vi "ZCAN_ReceiveData_2.vi"() -> ()   [LabVIEW 2020]
uses:
  data_type/ZCANDataObj.ctl
  bin/zlgcan_wrap.dll
panel:
  in  "type of receipt":enum16{"CAN", "CANFD", "合并接收"}(ring)=enum."合并接收"
  out "error out":errorcluster caption="错误输出"
  out "Receive_Num":u32
  in  "can_handle":u32
  in  "error in (no error)":errorcluster caption="错误输入（无错误）"
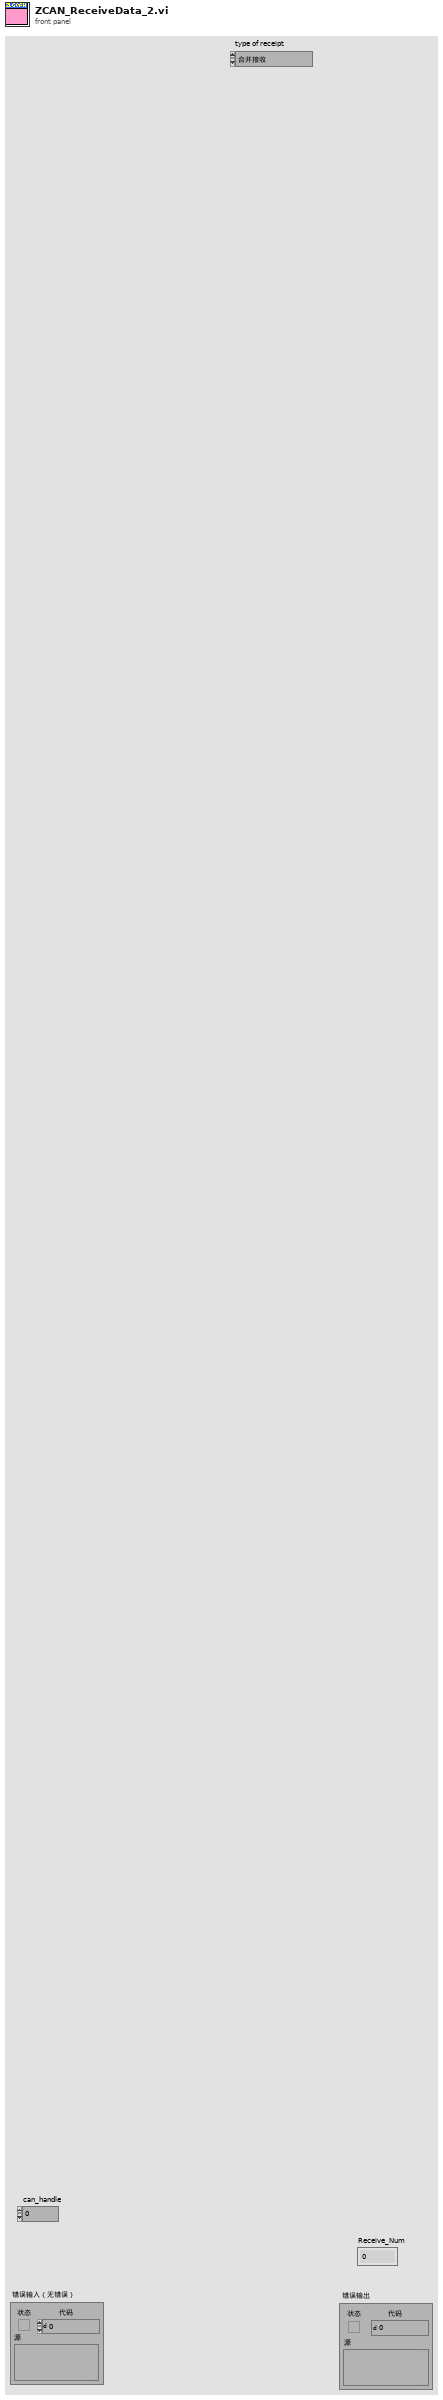
[diagram p1: front panel]
types:
  T1 = typedef "zlgcan.lvlib/ZCANDataObj.ctl" = cluster{"Data_Type":u8, "CAN_CH":u8, "rawVal(未使用)":u16, "extraData[4]（未使用）":cluster{"[0]":u8, "[1]":u8, "[2]":u8, "[3]":u8}, "canCANFDData":cluster{"时间戳+混合标志位":cluster{"时间戳":u64, "混合标志位":u32}, "extraData[4]（未使用）":cluster{"[0]":u8, "[1]":u8, "[2]":u8, "[3]":u8}, "frame":cluster{"can_id":u32, "Data长度":u8, "CANFD加速？":u8, "__res0":u8, "__res1":u8, "data":cluster{"CANData[0]":u8, "CANData[1]":u8, "CANData[2]":u8, "CANData[3]":u8, "CANData[4]":u8, "CANData[5]":u8, "CANData[6]":u8, "CANData[7]":u8, "CANData[8]":u8, "CANData[9]":u8, "CANData[10]":u8, "CANData[11] ":u8, "CANData[12] ":u8, "CANData[13] ":u8, "CANData[14] ":u8, "CANData[15] ":u8, "CANData[16]":u8, "CANData[17]":u8, "CANData[18]":u8, "CANData[19]":u8, "CANData[20]":u8, "CANData[21]":u8, "CANData[22]":u8, "CANData[23]":u8, "CANData[24] ":u8, "CANData[25]":u8, "CANData[26]":u8, "CANData[27]":u8, "CANData[28]":u8, "CANData[29]":u8, "CANData[30]":u8, "CANData[31]":u8, "CANData[32]":u8, "CANData[33]":u8, "CANData[34]":u8, "CANData[35]":u8, "CANData[36]":u8, "CANData[37]":u8, "CANData[38]":u8, "CANData[39]":u8, "CANData[40]":u8, "CANData[41]":u8, "CANData[42]":u8, "CANData[43]":u8, "CANData[44]":u8, "CANData[45]":u8, "CANData[46]":u8, "CANData[47]":u8, "CANData[48]":u8, "CANData[49]":u8, "CANData[50]":u8, "CANData[51]":u8, "CANData[52]":u8, "CANData[53]":u8, "CANData[54]":u8, "CANData[55]":u8, "CANData[56]":u8, "CANData[57]":u8, "CANData[58]":u8, "CANData[59]":u8, "CANData[60]":u8, "CANData[61]":u8, "CANData[62]":u8, "CANData[63]":u8}}}, "raw":cluster{"[0]":u8, "[1]":u8, "[2]":u8, "[3]":u8, "[4]":u8, "[5]":u8, "[6]":u8, "[7]":u8, "[8]":u8, "[9]":u8, "[10]":u8, "[11]":u8, "[12]":u8, "[13]":u8, "[14]":u8, "[15]":u8, "[16]":u8, "[17]":u8, "[18]":u8, "[19]":u8, "[20]":u8, "[21]":u8, "[22]":u8, "[23]":u8, "[24]":u8, "[25]":u8, "[26]":u8, "[27]":u8, "[28]":u8, "[29]":u8, "[30]":u8, "[31]":u8, "[32]":u8, "[33]":u8, "[34]":u8, "[35]":u8, "[36]":u8, "[37]":u8, "[38]":u8, "[39]":u8, "[40]":u8, "[41]":u8, "[42]":u8, "[43]":u8, "[44]":u8, "[45]":u8, "[46]":u8, "[47]":u8, "[48]":u8, "[49]":u8, "[50]":u8, "[51]":u8, "[52]":u8, "[53]":u8, "[54]":u8, "[55]":u8, "[56]":u8, "[57]":u8, "[58]":u8, "[59]":u8, "[60]":u8, "[61]":u8, "[62]":u8, "[63]":u8, "[64]":u8, "[65]":u8, "[73]":u8, "[72]":u8, "[71]":u8, "[70]":u8, "[69]":u8, "[68]":u8, "[67]":u8, "[66]":u8, "[74]":u8, "[75]":u8, "[83]":u8, "[82]":u8, "[81]":u8, "[80]":u8, "[79]":u8, "[78]":u8, "[77]":u8, "[76]":u8, "[84]":u8, "[85]":u8, "[91]":u8, "[90]":u8, "[89]":u8, "[88]":u8, "[87]":u8, "[86]":u8}}
  T2 = cluster{"时间戳+混合标志位":cluster{"时间戳":u64, "混合标志位":u32}, "extraData[4]（未使用）":cluster{"[0]":u8, "[1]":u8, "[2]":u8, "[3]":u8}, "frame":cluster{"can_id":u32, "Data长度":u8, "CANFD加速？":u8, "__res0":u8, "__res1":u8, "data":cluster{"CANData[0]":u8, "CANData[1]":u8, "CANData[2]":u8, "CANData[3]":u8, "CANData[4]":u8, "CANData[5]":u8, "CANData[6]":u8, "CANData[7]":u8, "CANData[8]":u8, "CANData[9]":u8, "CANData[10]":u8, "CANData[11] ":u8, "CANData[12] ":u8, "CANData[13] ":u8, "CANData[14] ":u8, "CANData[15] ":u8, "CANData[16]":u8, "CANData[17]":u8, "CANData[18]":u8, "CANData[19]":u8, "CANData[20]":u8, "CANData[21]":u8, "CANData[22]":u8, "CANData[23]":u8, "CANData[24] ":u8, "CANData[25]":u8, "CANData[26]":u8, "CANData[27]":u8, "CANData[28]":u8, "CANData[29]":u8, "CANData[30]":u8, "CANData[31]":u8, "CANData[32]":u8, "CANData[33]":u8, "CANData[34]":u8, "CANData[35]":u8, "CANData[36]":u8, "CANData[37]":u8, "CANData[38]":u8, "CANData[39]":u8, "CANData[40]":u8, "CANData[41]":u8, "CANData[42]":u8, "CANData[43]":u8, "CANData[44]":u8, "CANData[45]":u8, "CANData[46]":u8, "CANData[47]":u8, "CANData[48]":u8, "CANData[49]":u8, "CANData[50]":u8, "CANData[51]":u8, "CANData[52]":u8, "CANData[53]":u8, "CANData[54]":u8, "CANData[55]":u8, "CANData[56]":u8, "CANData[57]":u8, "CANData[58]":u8, "CANData[59]":u8, "CANData[60]":u8, "CANData[61]":u8, "CANData[62]":u8, "CANData[63]":u8}}}
  T3 = cluster{"can_id":u32, "Data长度":u8, "CANFD加速？":u8, "__res0":u8, "__res1":u8, "data":cluster{"CANData[0]":u8, "CANData[1]":u8, "CANData[2]":u8, "CANData[3]":u8, "CANData[4]":u8, "CANData[5]":u8, "CANData[6]":u8, "CANData[7]":u8, "CANData[8]":u8, "CANData[9]":u8, "CANData[10]":u8, "CANData[11] ":u8, "CANData[12] ":u8, "CANData[13] ":u8, "CANData[14] ":u8, "CANData[15] ":u8, "CANData[16]":u8, "CANData[17]":u8, "CANData[18]":u8, "CANData[19]":u8, "CANData[20]":u8, "CANData[21]":u8, "CANData[22]":u8, "CANData[23]":u8, "CANData[24] ":u8, "CANData[25]":u8, "CANData[26]":u8, "CANData[27]":u8, "CANData[28]":u8, "CANData[29]":u8, "CANData[30]":u8, "CANData[31]":u8, "CANData[32]":u8, "CANData[33]":u8, "CANData[34]":u8, "CANData[35]":u8, "CANData[36]":u8, "CANData[37]":u8, "CANData[38]":u8, "CANData[39]":u8, "CANData[40]":u8, "CANData[41]":u8, "CANData[42]":u8, "CANData[43]":u8, "CANData[44]":u8, "CANData[45]":u8, "CANData[46]":u8, "CANData[47]":u8, "CANData[48]":u8, "CANData[49]":u8, "CANData[50]":u8, "CANData[51]":u8, "CANData[52]":u8, "CANData[53]":u8, "CANData[54]":u8, "CANData[55]":u8, "CANData[56]":u8, "CANData[57]":u8, "CANData[58]":u8, "CANData[59]":u8, "CANData[60]":u8, "CANData[61]":u8, "CANData[62]":u8, "CANData[63]":u8}}
  T4 = cluster{"CANData[0]":u8, "CANData[1]":u8, "CANData[2]":u8, "CANData[3]":u8, "CANData[4]":u8, "CANData[5]":u8, "CANData[6]":u8, "CANData[7]":u8, "CANData[8]":u8, "CANData[9]":u8, "CANData[10]":u8, "CANData[11] ":u8, "CANData[12] ":u8, "CANData[13] ":u8, "CANData[14] ":u8, "CANData[15] ":u8, "CANData[16]":u8, "CANData[17]":u8, "CANData[18]":u8, "CANData[19]":u8, "CANData[20]":u8, "CANData[21]":u8, "CANData[22]":u8, "CANData[23]":u8, "CANData[24] ":u8, "CANData[25]":u8, "CANData[26]":u8, "CANData[27]":u8, "CANData[28]":u8, "CANData[29]":u8, "CANData[30]":u8, "CANData[31]":u8, "CANData[32]":u8, "CANData[33]":u8, "CANData[34]":u8, "CANData[35]":u8, "CANData[36]":u8, "CANData[37]":u8, "CANData[38]":u8, "CANData[39]":u8, "CANData[40]":u8, "CANData[41]":u8, "CANData[42]":u8, "CANData[43]":u8, "CANData[44]":u8, "CANData[45]":u8, "CANData[46]":u8, "CANData[47]":u8, "CANData[48]":u8, "CANData[49]":u8, "CANData[50]":u8, "CANData[51]":u8, "CANData[52]":u8, "CANData[53]":u8, "CANData[54]":u8, "CANData[55]":u8, "CANData[56]":u8, "CANData[57]":u8, "CANData[58]":u8, "CANData[59]":u8, "CANData[60]":u8, "CANData[61]":u8, "CANData[62]":u8, "CANData[63]":u8}
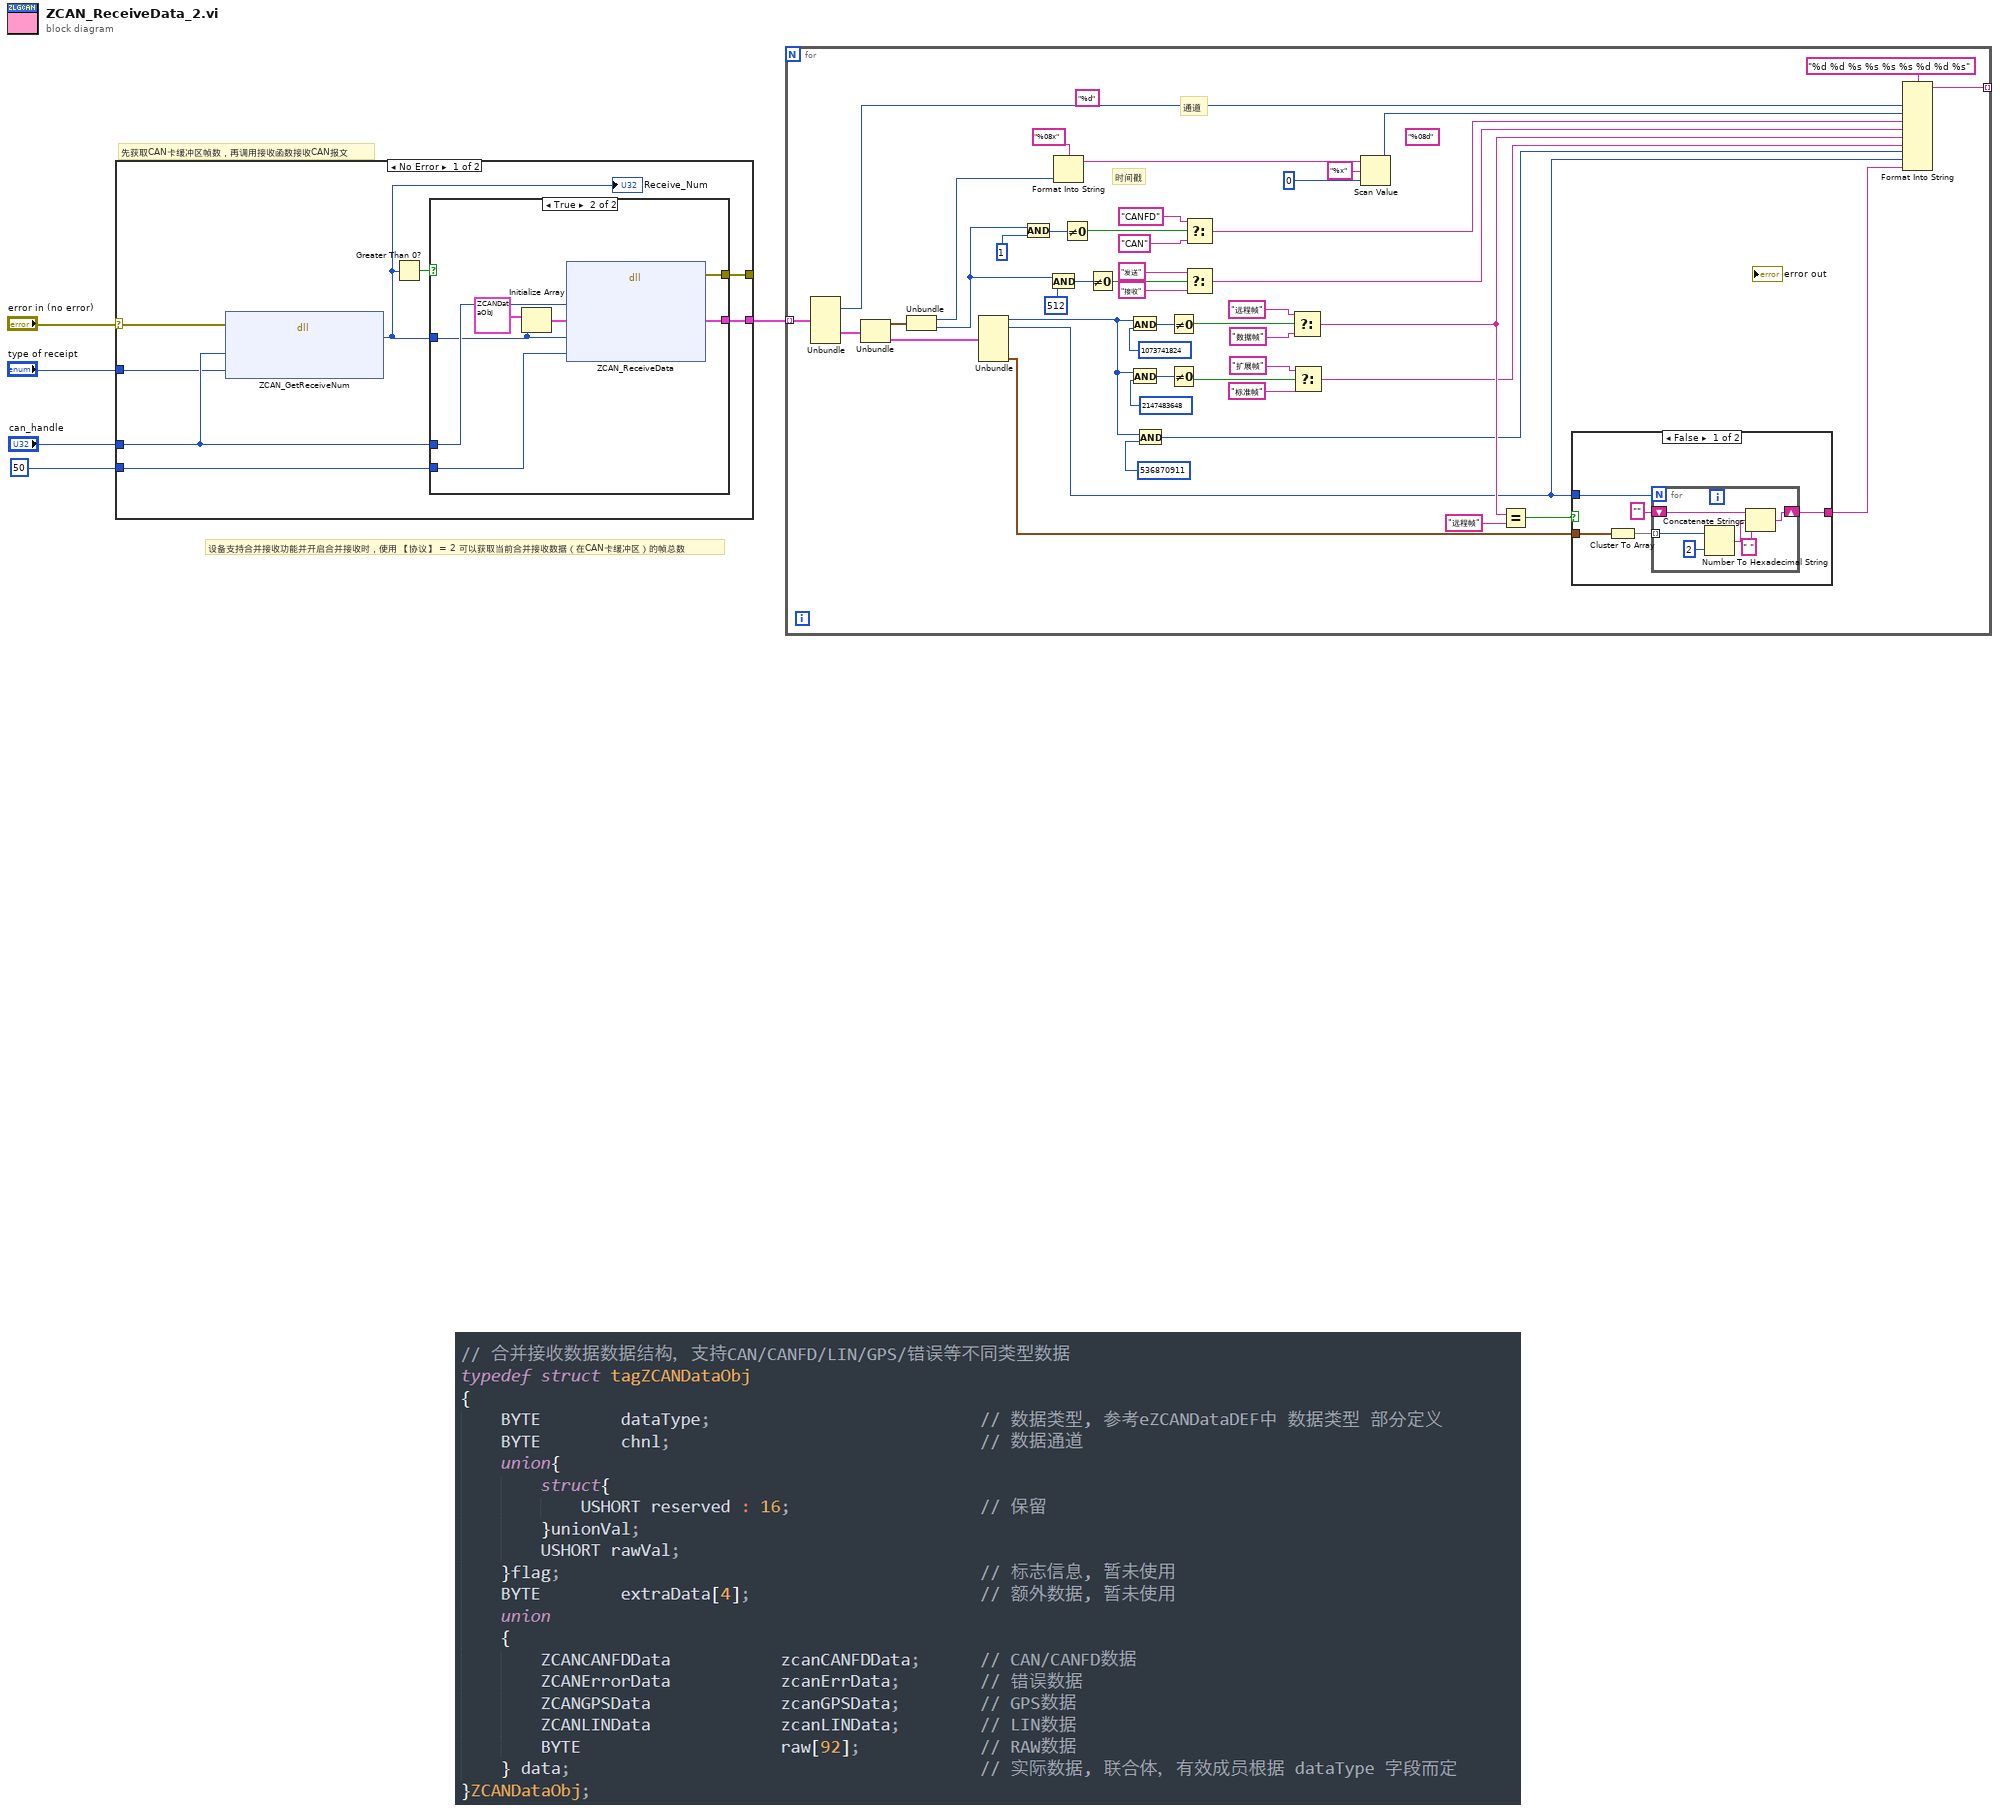
[diagram p0: block diagram]
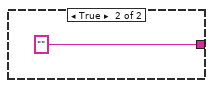
[diagram p2: hidden frame]
diagram:
  (unwired) "%d"
  # "先获取CAN卡缓冲区帧数，再调用接收函数接收CAN报文"
  # "设备支持合并接收功能并开启合并接收时，使用 【协议】 = 2 可以获取当前合并接收数据（在CAN卡缓冲区）的帧总数"
  n1 = case shown="No Error" "error in (no error)" {
    selector: "error in (no error)" -> [w13 _]
    tunnel: "can_handle" -> [w10 _]
    tunnel: [w11 _] -> w1
    tunnel: [w9 _] -> _
    tunnel: "type of receipt" -> [w8 _]
    tunnel: 50 ("超时时间") -> [w7 _]
    frame No Error {
      n2 = dll-call lib="D:/Git/ZLG_USBCANFD/bin/zlgcan_wrap.dll" fn="ZCAN_GetReceiveNum"(error in=w13, "通道句柄"=w10, "协议"=w8) -> ("缓冲区帧数"=w6:u32)  [unwired: 4 in, 2 out]
      "Receive_Num" <- w6
      n3 = Greater Than 0?(x=w6) -> (x > 0?=w12:bool)
      n4 = case shown="True" w12 {
        tunnel: w6 -> [_ w16]
        tunnel: [_ w20] -> w11
        tunnel: [_ w19] -> w9
        tunnel: w10 -> [_ w18]
        tunnel: w7 -> [_ w14]
        frame False {
        }
        frame True {
          n5 = Initialize Array(T1 {"Data_Type"=0, "CAN_CH"=0, "rawVal(未使用)"=0, "extraData[4]（未使用）"={"[0]"=0, "[1]"=0, "[2]"=0, "[3]"=0}, "canCANFDData"={"时间戳+混合标志位"={"时间戳"=0, "混合标志位"=0}, "extraData[4]（未使用）"={"[0]"=0, "[1]"=0, "[2]"=0, "[3]"=0}, "frame"={"can_id"=0, "Data长度"=0, "CANFD加速？"=0, "__res0"=0, "__res1"=0, "data"={"CANData[0]"=0, "CANData[1]"=0, "CANData[2]"=0, "CANData[3]"=0, "CANData[4]"=0, "CANData[5]"=0, "CANData[6]"=0, "CANData[7]"=0, "CANData[8]"=0, "CANData[9]"=0, "CANData[10]"=0, "CANData[11] "=0, "CANData[12] "=0, "CANData[13] "=0, "CANData[14] "=0, "CANData[15] "=0, "CANData[16]"=0, "CANData[17]"=0, "CANData[18]"=0, "CANData[19]"=0, "CANData[20]"=0, "CANData[21]"=0, "CANData[22]"=0, "CANData[23]"=0, "CANData[24] "=0, "CANData[25]"=0, "CANData[26]"=0, "CANData[27]"=0, "CANData[28]"=0, "CANData[29]"=0, "CANData[30]"=0, "CANData[31]"=0, "CANData[32]"=0, "CANData[33]"=0, "CANData[34]"=0, "CANData[35]"=0, "CANData[36]"=0, "CANData[37]"=0, "CANData[38]"=0, "CANData[39]"=0, "CANData[40]"=0, "CANData[41]"=0, "CANData[42]"=0, "CANData[43]"=0, "CANData[44]"=0, "CANData[45]"=0, "CANData[46]"=0, "CANData[47]"=0, "CANData[48]"=0, "CANData[49]"=0, "CANData[50]"=0, "CANData[51]"=0, "CANData[52]"=0, "CANData[53]"=0, "CANData[54]"=0, "CANData[55]"=0, "CANData[56]"=0, "CANData[57]"=0, "CANData[58]"=0, "CANData[59]"=0, "CANData[60]"=0, "CANData[61]"=0, "CANData[62]"=0, "CANData[63]"=0}}}, "raw"={"[0]"=0, "[1]"=0, "[2]"=0, "[3]"=0, "[4]"=0, "[5]"=0, "[6]"=0, "[7]"=0, "[8]"=0, "[9]"=0, "[10]"=0, "[11]"=0, "[12]"=0, "[13]"=0, "[14]"=0, "[15]"=0, "[16]"=0, "[17]"=0, "[18]"=0, "[19]"=0, "[20]"=0, "[21]"=0, "[22]"=0, "[23]"=0, "[24]"=0, "[25]"=0, "[26]"=0, "[27]"=0, "[28]"=0, "[29]"=0, "[30]"=0, "[31]"=0, "[32]"=0, "[33]"=0, "[34]"=0, "[35]"=0, "[36]"=0, "[37]"=0, "[38]"=0, "[39]"=0, "[40]"=0, "[41]"=0, "[42]"=0, "[43]"=0, "[44]"=0, "[45]"=0, "[46]"=0, "[47]"=0, "[48]"=0, "[49]"=0, "[50]"=0, "[51]"=0, "[52]"=0, "[53]"=0, "[54]"=0, "[55]"=0, "[56]"=0, "[57]"=0, "[58]"=0, "[59]"=0, "[60]"=0, "[61]"=0, "[62]"=0, "[63]"=0, "[64]"=0, "[65]"=0, "[73]"=0, "[72]"=0, "[71]"=0, "[70]"=0, "[69]"=0, "[68]"=0, "[67]"=0, "[66]"=0, "[74]"=0, "[75]"=0, "[83]"=0, "[82]"=0, "[81]"=0, "[80]"=0, "[79]"=0, "[78]"=0, "[77]"=0, "[76]"=0, "[84]"=0, "[85]"=0, "[91]"=0, "[90]"=0, "[89]"=0, "[88]"=0, "[87]"=0, "[86]"=0}} ("ZCANDataObj"), w16) -> (w15:T1[])
          n6 = dll-call lib="D:/Git/ZLG_USBCANFD/bin/zlgcan_wrap.dll" fn="ZCAN_ReceiveData"("通道句柄"=w18, "数据帧数组"=w15, "数据帧数"=w16, "超时时间"=w14) -> (error out=w19:errorcluster, "数据帧数组"=w20:T1[])  [unwired: 7 in, 1 out]
        }
      }
    }
    frame Error {
    }
  }
  n7 = for {
    tunnel: w1 -> [w54] mode=indexing
    tunnel: [w22] -> _ mode=indexing
    (unwired) "%08d"
    # "时间戳"
    # "通道"
    n8 = Unbundle(w54) -> ("CAN_CH"=w23:u8, "canCANFDData"=w35:T2)  [unwired: 4 out]
    n9 = Unbundle(w35) -> ("时间戳+混合标志位"=w53:cluster{"时间戳":u64, "混合标志位":u32}, "frame"=w34:T3)  [unwired: 1 out]
    n10 = Unbundle(w53) -> ("时间戳"=w39:u64, "混合标志位"=w41:u32)
    n11 = Unbundle(w34) -> ("can_id"=w40:u32, "Data长度"=w28:u8, "data"=w25:T4)  [unwired: 3 out]
    n12 = And(x=w41, y=u32 1) -> (x .and. y?=w50:u32)
    n13 = And(x=w41, y=u32 512) -> (x .and. y?=w45:u32)
    n14 = Format Into String(format string="%08x", w39) -> (resulting string=w38:string)  [unwired: 2 in, 1 out]
    n15 = Not Equal To 0?(x=w50) -> (x != 0?=w47:bool)
    n16 = Not Equal To 0?(x=w45) -> (x != 0?=w42:bool)
    n17 = And(x=w40, y=u32 1073741824) -> (x .and. y?=w62:u32)
    n18 = And(x=w40, y=u32 2147483648) -> (x .and. y?=w63:u32)
    n19 = And(x=w40, y=u32 536870911) -> (x .and. y?=w29:u32)
    n20 = Not Equal To 0?(x=w62) -> (x != 0?=w57:bool)
    n21 = Not Equal To 0?(x=w63) -> (x != 0?=w56:bool)
    n22 = Select(t="CANFD", s=w47, f="CAN") -> (s? t:f=w33:string)
    n23 = Select(t="发送", s=w42, f="接收") -> (s? t:f=w32:string)
    n24 = Select(t="远程帧", s=w57, f="数据帧") -> (s? t:f=w31:string)
    n25 = Select(t="扩展帧", s=w56, f="标准帧") -> (s? t:f=w30:string)
    n26 = Scan Value(string=w38, format string="%x", default (0 dbl)=0) -> (value=w24:i32)  [unwired: 1 out]
    n27 = Equal?(x=w31, y="远程帧") -> (x = y?=w26:bool)
    n28 = case shown="False" w26 {
      tunnel: w28 -> [w70 _]
      tunnel: [w69 ""] -> w27
      tunnel: w25 -> [w68 _]
      frame False {
        n29 = Cluster To Array(cluster=w68) -> (array=w67:u8[])
        n30 = for {
          N: w70 -> [_]
          shift-right: [w74] -> w69
          shift-left: "" -> [w72]
          tunnel: w67 -> [w73] mode=indexing
          n31 = Number To Hexadecimal String(1:i16 2 ("width (-)"), 2:w73) -> (0:w76:string)
          n32 = Concatenate Strings(w72, w76, " " ("string")) -> (w74:string)
        }
      }
      frame True {
      }
    }
    n33 = Format Into String(format string="%d %d %s %s %s %s %d %d %s", w23, w24, w33, w32, w31, w30, w29, w28, w27) -> (resulting string=w22:string)  [unwired: 2 in, 1 out]
  }
